vi "Clear Error 1149.vi"(8 "error in (no error)":errorcluster) -> (0 "error out":errorcluster)   [LabVIEW 2020, in "Error Manager.lvlib"]
doc: "Blank VI with error handling."
uses:
  Error Manager.lvlib
panel:
  # "Development\ncontrols/indicators useful for development and testing, but which are not outputs of the VI"
  # "Input\nInputs to the VI"
  # "Output\nOutputs of the VI"
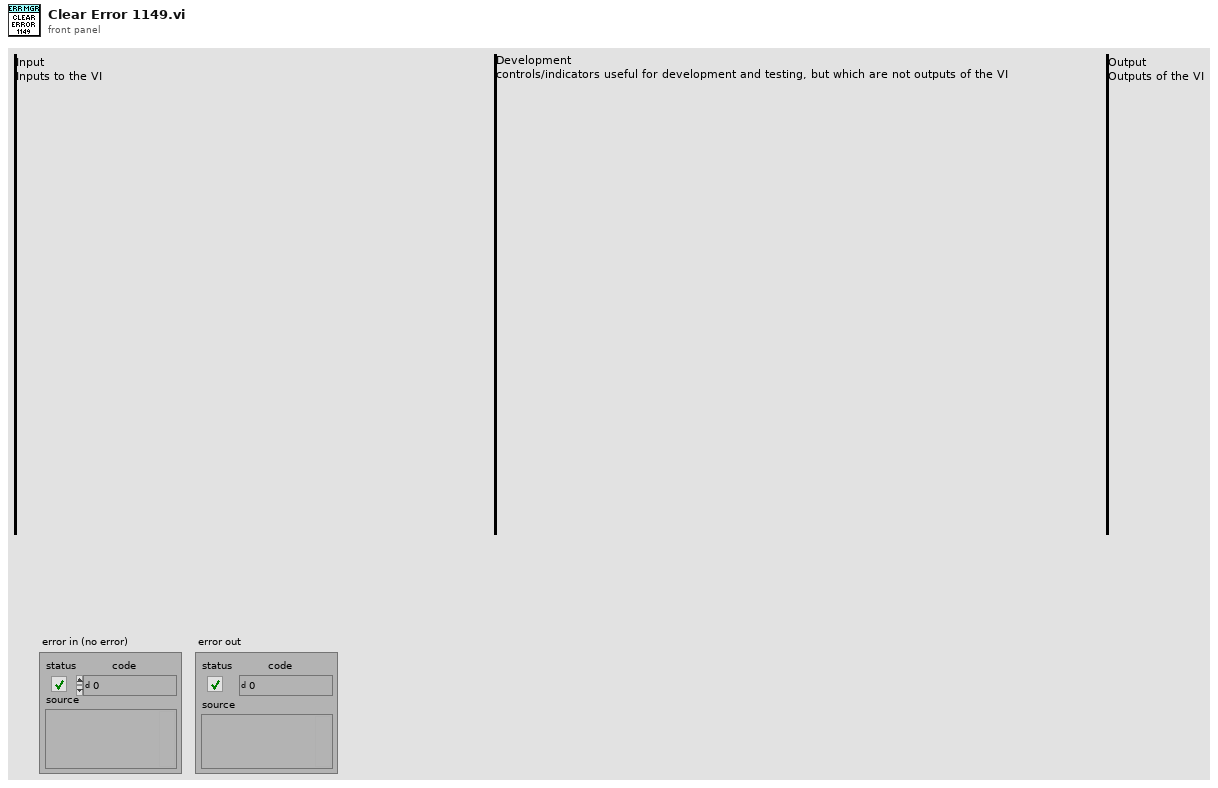
[diagram p1: front panel]
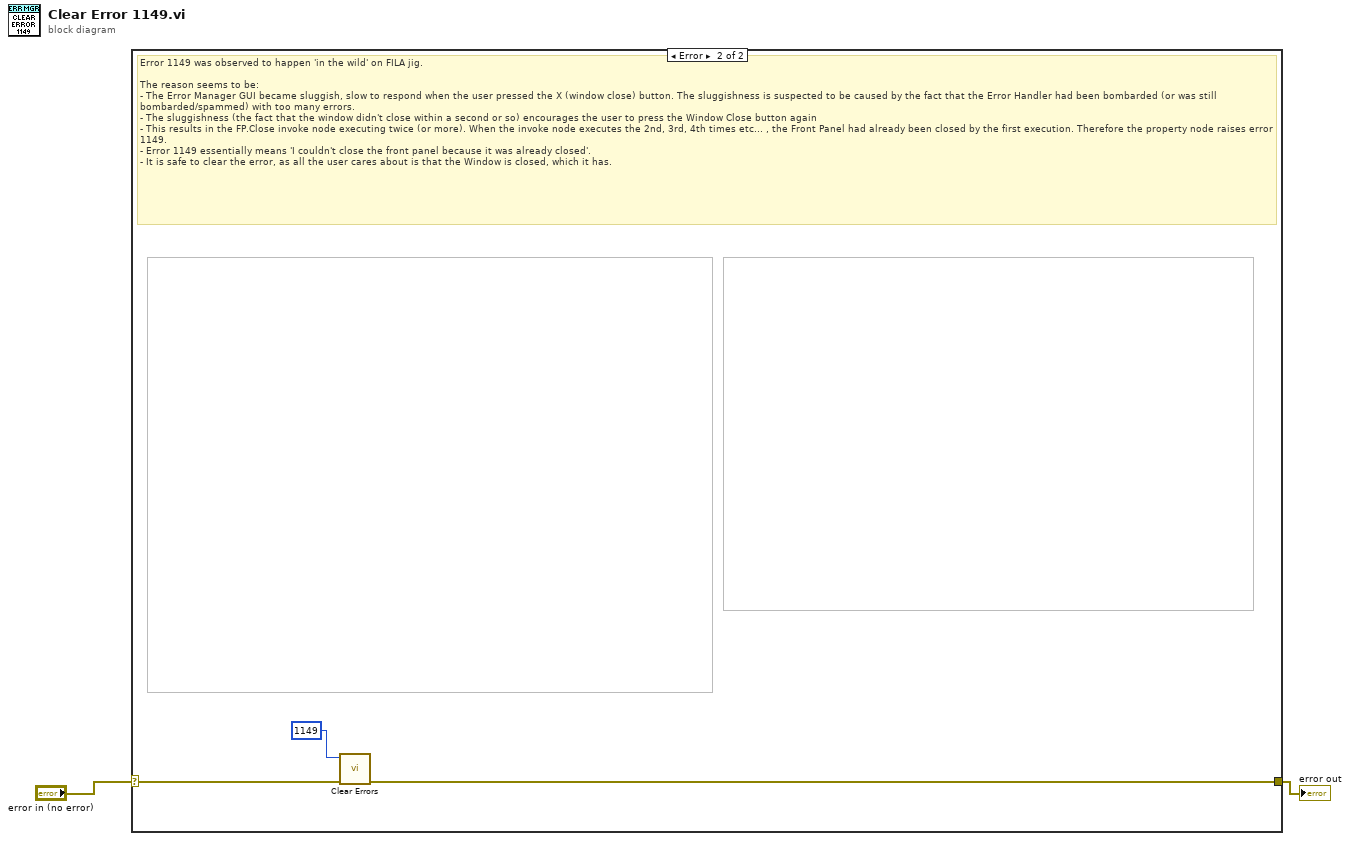
[diagram p0: block diagram]
diagram:
  n1 = case shown="Error" "error in (no error)" {
    selector: "error in (no error)" -> [w3 w6]
    tunnel: [w3 w5] -> w1
    frame No Error {
      # "This case expected to execute most of the time. Do nothing."
    }
    frame Error {
      # "Error 1149 was observed to happen 'in the wild' on FILA jig.\n\nThe reason seems to be:\n- The Error Manager GUI became sluggish, slow to respond when the user pressed the X (window close) button. The sluggishness is suspected to be caused by the fact that the Error Handler had been bombarded (or was still bombarded/spammed) with too many errors.\n- The sluggishness (the fact that the window didn't close within a second or so) encourages the user to press the Window Close button again\n- This results in the FP.Close invoke node executing twice (or more). When the invoke node executes the 2nd, 3rd, 4th times etc... , the Front Panel had already been closed by the first execution. Therefore the property node raises error 1149.\n- Error 1149 essentially means 'I couldn't close the front panel because it was already closed'.\n- It is safe to clear the error, as all the user cares about is that the Window is closed, which it has."
      n2 = call <vilib>:"Clear Errors.vi"("error in (no error)"=w6, "specific error code to clear (0: all)"=1149) -> ("error out"=w5:errorcluster)  [unwired: 4 in, 1 out]
    }
  }
  "error out" <- w1
